vi "pedFile.vi"(4 "pattern":string="/u2/data/btf/data/") -> (1 "last Ped File":path)   [LabVIEW 2014]
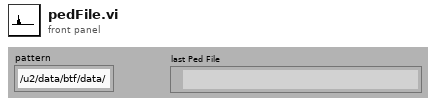
[diagram p1: front panel]
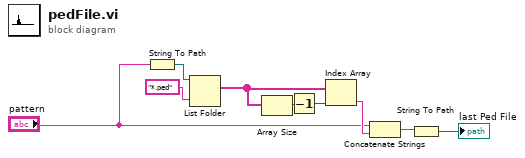
[diagram p0: block diagram]
diagram:
  n1 = String To Path(string="pattern") -> (path=w2:path)
  n2 = List Folder(path=w2, pattern="*.ped") -> (filenames=w9:string[])  [unwired: 2 in, 3 out]
  n3 = Array Size(array=w9) -> (size(s)=w8:i32)
  n4 = Decrement(x=w8) -> (x-1=w7:i32)
  n5 = Index Array(array=w9, index=w7) -> (element=w6:string)
  n6 = Concatenate Strings("pattern", w6) -> (w5:string)
  n7 = String To Path(string=w5) -> (path=→"last Ped File":path)
